vi "Insert Results into Excel.vi"(0 "report in":refnum<class "NI_report.lvclass">, 1 "strings":string[](array[string]), 2 "Pass/Fail":bool[](array[boolean]), 5 "column":i32, 7 "row":i32, 11 "error in":errorcluster) -> (4 "report out":refnum<class "NI_report.lvclass">, 6 "column out":i32, 15 "error out":errorcluster)   [LabVIEW 2015]
uses:
  <vilib>/Utility/NIReport.llb/NI_report.lvclass
  <vilib>/Utility/NIReport.llb/Append Report Text (str wrap).vi
  <vilib>/Utility/NIReport.llb/Excel/NI_Excel.lvclass
panel:
  in  "outside border":T1={"on/off"=TRUE, "weight"=2, "color"=7631988} {"weight" items=["xlHairline"=1, "xlMedium"=-4138, "xlThick"=4, "xlThin"=2]}
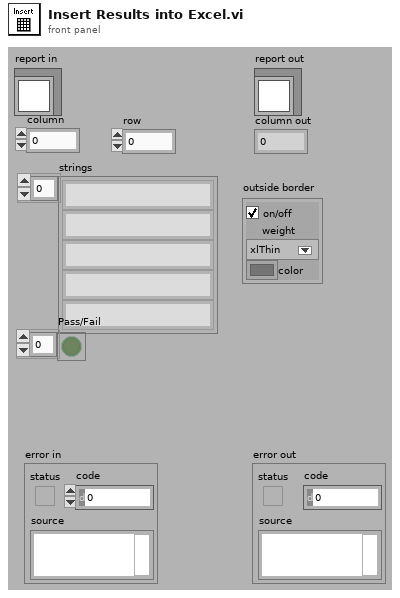
[diagram p1: front panel]
types:
  T1 = cluster{"on/off":bool, "weight":i32, "color":u32}
  T2 = cluster{"position (excel)":cluster{"row":i32, "column":i32}, "name (excel)":string, "bookmark (word)":string}
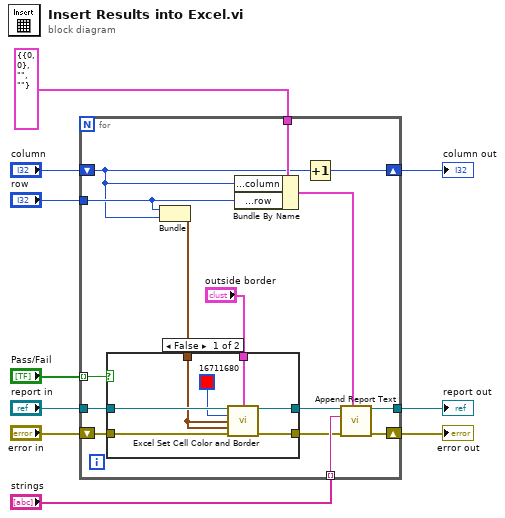
[diagram p0: block diagram]
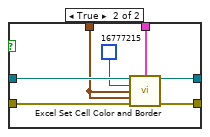
[diagram p2: hidden frame]
diagram:
  n1 = for {
    tunnel: "strings" -> [w25] mode=indexing
    tunnel: "report in" -> [w12]
    tunnel: [w24] -> w2
    shift-right: [w20] -> w5
    shift-left: "column" -> [w14]
    tunnel: T2 {"position (excel)"={"row"=0, "column"=0}, "name (excel)"="", "bookmark (word)"=""} ("MS Office parameters") -> [w22]
    tunnel: "row" -> [w17]
    shift-right: [w23] -> w1
    shift-left: "error in" -> [w13]
    tunnel: "Pass/Fail" -> [w15] mode=indexing
    n2 = Bundle("row"=w17, "column"=w14) -> (w16:cluster{"row":i32, "column":i32})  [unwired: 1 in]
    n3 = case shown="False" w15 {
      tunnel: [w32 w39] -> w19
      tunnel: [w31 w38] -> w18
      tunnel: w12 -> [w30 w37]
      tunnel: w13 -> [w29 w36]
      tunnel: w16 -> [w28 w35]
      tunnel: "outside border" -> [w26 w33]
      frame False {
        n4 = call <vilib>:"Excel Set Cell Color and Border.vi"("report in"=w30, "outside border"=w26, "background color (w)"=u32 16711680, "start (-1, -1)"=w28, "end (-1, -1)"=w28, "error in (no error)"=w29) -> ("report out"=w32:refnum<class "NI_report.lvclass">, "error out"=w31:errorcluster)  [unwired: 8 in]
      }
      frame True {
        n5 = call <vilib>:"Excel Set Cell Color and Border.vi"("report in"=w37, "outside border"=w33, "background color (w)"=u32 16777215, "start (-1, -1)"=w35, "end (-1, -1)"=w35, "error in (no error)"=w36) -> ("report out"=w39:refnum<class "NI_report.lvclass">, "error out"=w38:errorcluster)  [unwired: 8 in]
      }
    }
    n6 = Bundle By Name(cluster=w22, "position (excel).column"=w14, "position (excel).row"=w17) -> (w21:T2)
    n7 = Increment(x=w14) -> (x+1=w20:i32)
    n8 = call-poly <vilib>:"Append Report Text.vi"("report in"=w19, "MS Office parameters"=w21, "text"=w25, "error in (no error)"=w18) -> ("report out"=w24:refnum<class "NI_report.lvclass">, "error out"=w23:errorcluster)  [unwired: 8 in, 2 out]
  }
  "error out" <- w1
  "column out" <- w5
  "report out" <- w2
